vi "Configure Totalize Gate.vi"(7 "Totalize Gate Polarity (1: Negative)":i32(ring)=1 items=["Positive", "Negative"], 8 "error in (no error)":errorcluster, 9 "Totalize Gate Time (0.1 s)":dbl=0.1, 10 "Totalize Gate Source (0: Time)":i32(ring) items=["Time", "External", "Input1", "Input2", "Advanced"], 11 "VISA resource name":refnum<visa-resource-name>) -> (0 "error out":errorcluster, 3 "VISA resource name out":refnum<visa-resource-name>)   [LabVIEW 2021, in "Agilent 532XX Series.lvlib"]
doc: "Configures the characteristics of time totalize gate.\n\n<B>Note:</B> This VI only applies to the Agilent 53220A/53230A."
uses:
  <instrlib>/Agilent 532XX Series/Agilent 532XX Series.lvlib
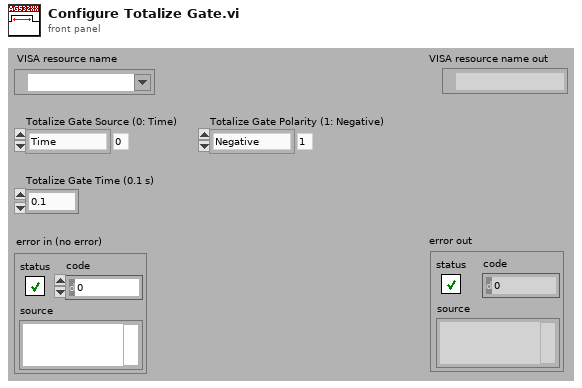
[diagram p1: front panel]
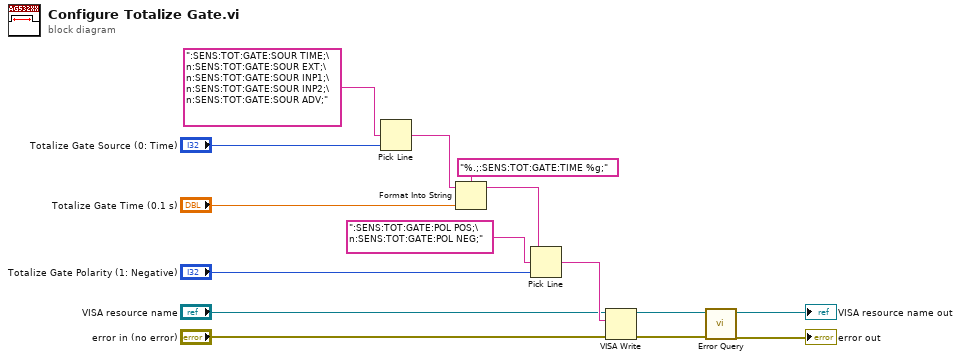
[diagram p0: block diagram]
diagram:
  n1 = Pick Line(multi-line string=":SENS:TOT:GATE:SOUR TIME;\n:SENS:TOT:GATE:SOUR EXT;\n:SENS:TOT:GATE:SOUR INP1;\n:SENS:TOT:GATE:SOUR INP2;\n:SENS:TOT:GATE:SOUR ADV;", line index="Totalize Gate Source (0: Time)") -> (output string=w13:string)  [unwired: 1 out]
  n2 = Format Into String(format string="%.;:SENS:TOT:GATE:TIME %g;", initial string=w13, "Totalize Gate Time (0.1 s)") -> (resulting string=w8:string)  [unwired: 1 in, 1 out]
  n3 = Pick Line(string ("")=w8, multi-line string=":SENS:TOT:GATE:POL POS;\n:SENS:TOT:GATE:POL NEG;", line index="Totalize Gate Polarity (1: Negative)") -> (output string=w7:string)
  n4 = VISA Write(VISA resource name="VISA resource name", write buffer=w7, error in (no error)="error in (no error)") -> (VISA resource name out=w4:refnum<visa-resource-name>, error out=w3:errorcluster)  [unwired: 1 out]
  n5 = call <instrlib>:"Error Query.vi"("error in (no error)"=w3, "VISA resource name"=w4) -> ("error out"=→"error out":errorcluster, "VISA resource name out"=→"VISA resource name out":refnum<visa-resource-name>)  [unwired: 8 out]
